vi "Open.vi"(6 "File Extension":string="csv", 7 "Start Time Stamp":timestamp, 8 "Error In":errorcluster, 10 "Enable Calendar Tree":bool=TRUE, 11 "Base Folder":path) -> (0 "Error Out":errorcluster, 3 "Log Out":refnum<file>)   [LabVIEW 2015, in "Logger.lvlib" / "File.lvlib"]
uses:
  File.lvlib
  <vilib>/Utility/libraryn.llb/Check if File or Folder Exists.vi
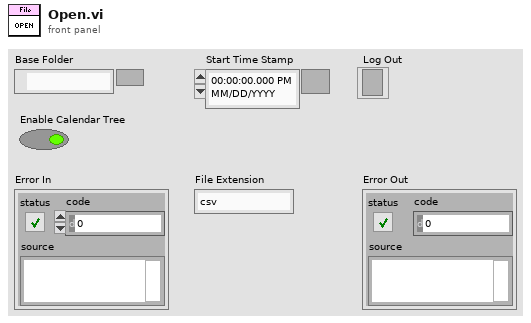
[diagram p1: front panel]
types:
  T1 = enum16{"open", "replace", "create", "open or create", "replace or create", "replace or create with confirmation"}
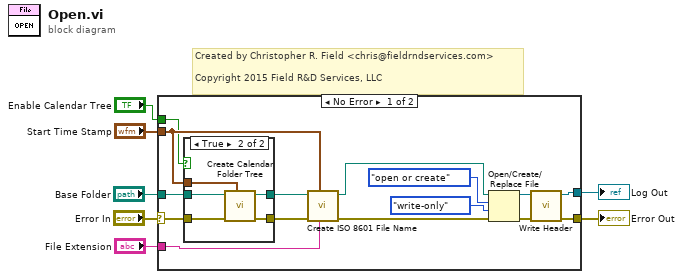
[diagram p0: block diagram]
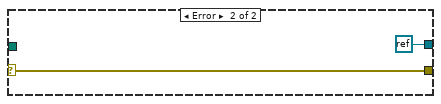
[diagram p3: hidden frame]
diagram:
  # "Created by Christopher R. Field <chris@fieldrndservices.com>\n\nCopyright 2015 Field R&D Services, LLC"
  n1 = case shown="No Error" "Error In" {
    selector: "Error In" -> [w19 w31]
    tunnel: "Base Folder" -> [w20 _]
    tunnel: "Start Time Stamp" -> [w16 _]
    tunnel: [w10 refnum<k0> refnum] -> w4
    tunnel: [w9 w31] -> w3
    tunnel: "Enable Calendar Tree" -> [w11 _]
    tunnel: "File Extension" -> [w8 _]
    frame No Error {
      n2 = case shown="True" w11 {
        tunnel: w20 -> [w24 w29]
        tunnel: w19 -> [w23 w28]
        tunnel: [w24 w27] -> w18
        tunnel: [w23 w26] -> w17
        tunnel: w16 -> [_ w25]
        frame False {
        }
        frame True {
          n3 = call "Create Calendar Folder Tree.vi"("Start Time Stamp"=w25, "Error In"=w28, "Base Log Folder"=w29) -> ("Error Out"=w26:errorcluster, "Calendar Folder Tree"=w27:path)  [unwired: 7 in]
        }
      }
      n4 = call "Create ISO 8601 File Name.vi"("File Extension"=w8, "Start Time Stamp"=w16, "Error In"=w17, "Log Folder"=w18) -> ("Error Out"=w14:errorcluster, "ISO 8601 File"=w15:path)  [unwired: 6 in]
      n5 = Open/Create/Replace File(file path (use dialog)=w15, error in=w14, operation (0:open)=T1."open or create", access (0:read/write)=enum16{"read/write", "read-only", "write-only"}."write-only") -> (refnum out=w13:refnum<file>, error out=w12:errorcluster)  [unwired: 2 in, 1 out]
      n6 = call "Write Header.vi"("Error In"=w12, "Log In"=w13) -> ("Error Out"=w9:errorcluster, "Log Out"=w10:refnum<file>)  [unwired: 8 in]
    }
    frame Error {
    }
  }
  "Log Out" <- w4
  "Error Out" <- w3
